vi "NT Change Client Mode.vi"(11 "Local":bool) -> ()   [LabVIEW 2025]
uses:
  ntcoreffi.dll
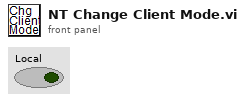
[diagram p1: front panel]
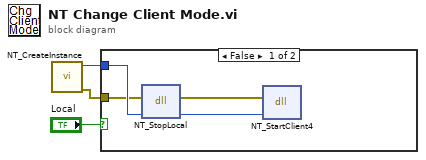
[diagram p0: block diagram]
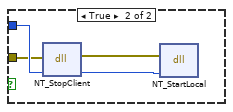
[diagram p2: hidden frame]
diagram:
  n1 = call <vilib>:"NT_CreateInstance.vi"() -> ("error out"=w1:errorcluster, "InstanceHandle"=w3:u64)  [unwired: 10 in]
  n2 = case shown="False" "Local" {
    tunnel: w3 -> [w6 w10]
    tunnel: w1 -> [w4 w8]
    frame False {
      n3 = dll-call lib="ntcoreffi.*" fn="NT_StopLocal"(error in=w4, "InstHandle"=w6) -> (error out=w7:errorcluster, "InstHandle"=w5:u64)  [unwired: 3 in, 1 out]
      n4 = dll-call lib="ntcoreffi.*" fn="NT_StartClient4"(error in=w7, "InstHandle"=w5) -> ()  [unwired: 4 in, 2 out]
    }
    frame True {
      n5 = dll-call lib="ntcoreffi.*" fn="NT_StopClient"(error in=w8, "InstHandle"=w10) -> (error out=w11:errorcluster, "InstHandle"=w9:u64)  [unwired: 3 in, 1 out]
      n6 = dll-call lib="ntcoreffi.*" fn="NT_StartLocal"(error in=w11, "InstHandle"=w9) -> ()  [unwired: 4 in, 2 out]
    }
  }
